vi "example_multipleRun_stopNotifier.vi"() -> ()   [LabVIEW 2023]
doc: "TLC Daemon Example Multiple Run - Boolean Stop Notifier"
uses:
  ExampleTask_StopNotifier/ExampleTask_BoolStopNotifier.lvclass
  TaskController/TaskController.lvclass
panel:
  out "loopCounter":i32[](array[numeric])
  out "isRunning":bool[](array[boolean])
  # "Example of Boolean Notifier Stop Mechanism"
  # "Instruction:\n1. Press RUN button.\n\n2. 10 tasks will run for approximately 5 seconds and then stop:\n    - the isRunning leds will be True during task execution.\n    - the loopCounter fields shows loopCounter value taken from the task outputs. \n\nFor details, view code and its comments"
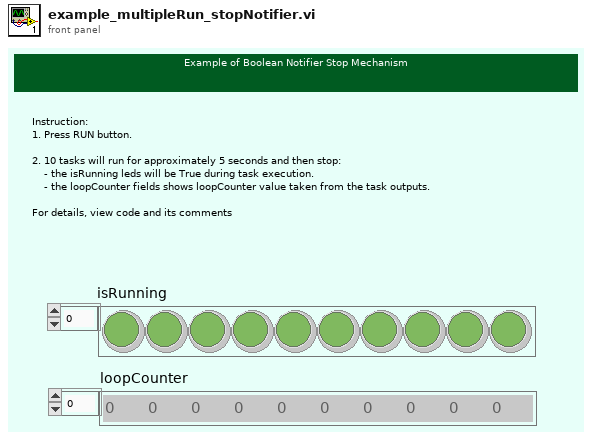
[diagram p1: front panel]
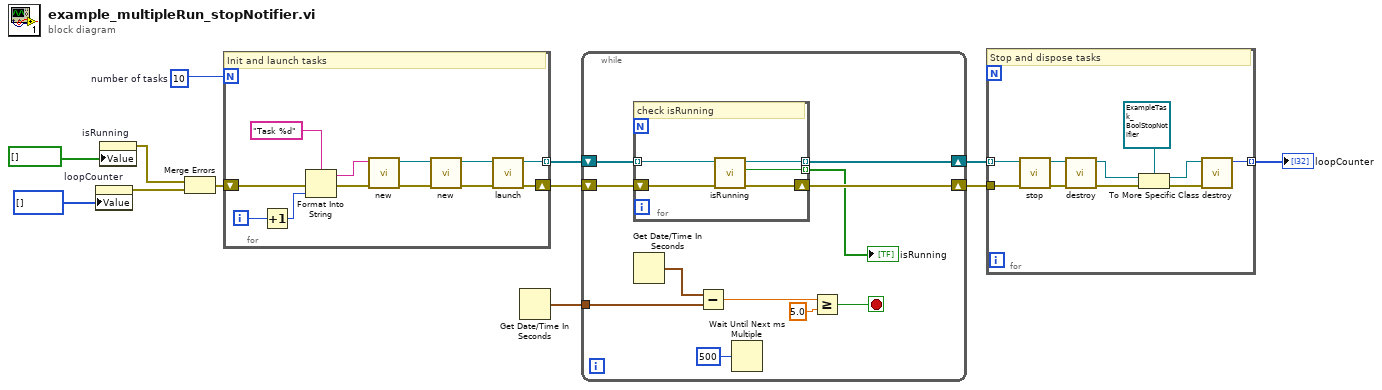
[diagram p0: block diagram]
diagram:
  w2 = 10  # number of tasks
  n1 = property on="loopCounter" class="Arr (strict)"("Value"=i32[] [] ("loopCounter")) -> (error out=w7:errorcluster)  [unwired: 2 in, 1 out]
  n2 = property on="isRunning" class="Arr (strict)"("Value"=bool[] [] ("isRunning")) -> (error out=w6:errorcluster)  [unwired: 2 in, 1 out]
  n3 = Merge Errors(w6, w7) -> (w5:errorcluster)
  n4 = for {
    N: w2 -> [_]
    tunnel: [w20] -> w11 mode=indexing
    shift-right: [w21] -> w12
    shift-left: w5 -> [w14]
    i -> [w18]
    # "Init and launch tasks"
    n5 = Increment(x=w18) -> (x+1=w17:i32)
    n6 = Format Into String(format string="Task %d", error in=w14, w17) -> (resulting string=w15:string, error out=w13:errorcluster)  [unwired: 1 in]
    n7 = call "new.vi"("error in (no error)"=w13, "description"=w15) -> ("error out"=w24:errorcluster, "ExampleTask_StopNotifier out"=w19:refnum<class "ExampleTask_BoolStopNotifier.lvclass">)  [unwired: 8 in]
    n8 = call "new.vi"("error in (no error)"=w24, "task"=w19) -> ("error out"=w23:errorcluster, "TaskController out"=w22:refnum<class "TaskController.lvclass">)  [unwired: 8 in]
    n9 = call "launch.vi"("error in (no error)"=w23, "TaskController in"=w22) -> ("error out"=w21:errorcluster, "TaskController out"=w20:refnum<class "TaskController.lvclass">)  [unwired: 8 in]
  }
  n10 = Get Date/Time In Seconds() -> (seconds since 1Jan1904=w1:timestamp)
  n11 = while {
    shift-right: [w33] -> w9
    shift-left: w11 -> [w34]
    shift-right: [w32] -> w10
    shift-left: w12 -> [w35]
    tunnel: w1 -> [w28]
    stop <- w25 stop-if-true
    n12 = for {
      tunnel: w34 -> [w39] mode=indexing
      tunnel: [w38] -> w33 mode=indexing
      shift-right: [w37] -> w32
      shift-left: w35 -> [w40]
      tunnel: [w36] -> w30 mode=indexing
      # "check isRunning"
      n13 = call "isRunning.vi"("error in (no error)"=w40, "TaskController in"=w39) -> ("error out"=w37:errorcluster, "isRunning"=w36:bool, "TaskController out"=w38:refnum<class "TaskController.lvclass">)  [unwired: 7 in]
    }
    "isRunning" <- w30
    n14 = Get Date/Time In Seconds() -> (seconds since 1Jan1904=w29:timestamp)
    n15 = Subtract(x=w29, y=w28) -> (x-y=w27:dbl)
    n16 = Wait Until Next ms Multiple(millisecond multiple=u32 500 ("milliseconds to wait")) -> ()  [unwired: 1 out]
    n17 = Greater Or Equal?(x=w27, y=5.0) -> (x >= y?=w25:bool)
  }
  n18 = for {
    tunnel: w10 -> [w50]
    tunnel: w9 -> [w49] mode=indexing
    tunnel: [w44] -> w8 mode=indexing
    # "Stop and dispose tasks"
    n19 = call "stop.vi"("error in (no error)"=w50, "TaskController in"=w49) -> ("error out"=w41:errorcluster, "TaskController out"=w42:refnum<class "TaskController.lvclass">)  [unwired: 8 in]
    n20 = call "destroy.vi"("error in (no error)"=w41, "TaskController in"=w42) -> ("error out"=w47:errorcluster, "taskResult"=w48:refnum<class "ITask.lvclass">)  [unwired: 7 in, 1 out]
    n21 = To More Specific Class(target class=refnum<class "ExampleTask_BoolStopNotifier.lvclass"> refnum ("ExampleTask_StopNotifier out"), reference=w48, error in=w47) -> (specific class reference=w46:refnum<class "ExampleTask_BoolStopNotifier.lvclass">, error out=w45:errorcluster)
    n22 = call "destroy.vi"("error in (no error)"=w45, "ExampleTask_StopNotifier in"=w46) -> ("loopCounter"=w44:i32)  [unwired: 8 in, 1 out]
  }
  "loopCounter" <- w8
